vi "Delete Storage Wrapper.vi"(8 "error in (no error)":errorcluster, 10 "key":string="myhome/kitchen/temp", 11 "Session in":u64) -> (0 "error out":errorcluster)   [LabVIEW 2021, in "Zenoh.lvclass"]
uses:
  Zenoh.lvclass
  Zenoh.lvclass/Zenoh.ctl
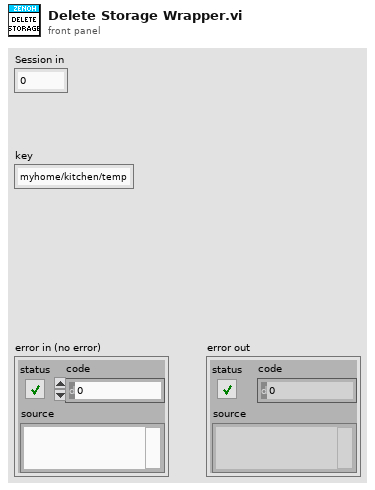
[diagram p1: front panel]
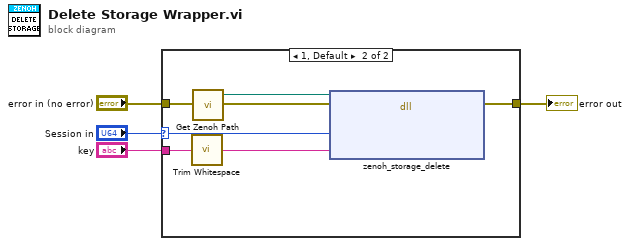
[diagram p0: block diagram]
diagram:
  n1 = case shown="1, Default" "Session in" {
    selector: "Session in" -> [_ w9]
    tunnel: [w5 w7] -> w4
    tunnel: "error in (no error)" -> [w5 w10]
    tunnel: "key" -> [_ w8]
    frame 0 {
    }
    frame 1, Default {
      n2 = call <vilib>:"Trim Whitespace.vi"("string"=w8) -> ("trimmed string"=w6:string)  [unwired: 1 in]
      n3 = call "Get Zenoh Path.vi"() -> ("Library Path"=w11:path)  [unwired: 4 in]
      n4 = dll-call lib="C:/Program Files/CIF_Foundation/Libraries/zenoh_lv_wrapper.dll" fn="zenoh_storage_delete"(path in=w11, error in=w10, "session_ptr"=w9, "key"=w6) -> (error out=w7:errorcluster)  [unwired: 4 in, 1 out]
    }
  }
  "error out" <- w4
